vi "SVT Spurious Free Dynamic Range.vi"   [LabVIEW 2017, in "SoundVib_SingleTone.lvlib"]
doc: "Computes the spurious-free dynamic range (SFDR) of <B>scaled signal</B> and returns the detected fundamental frequency, detected fundamental amplitude, spurious free dynamic range, and all detected peaks. Wire data to the <B>scaled signal [EU]</B> input to determine the polymorphic instance to use or manually select the instance."
uses:
  <vilib>/addons/Sound and Vibration/svt_Single Tone Measurements/SoundVib_SingleTone.lvlib
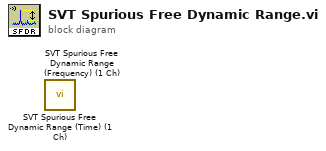
[diagram p0: block diagram]
diagram:
  n1 = call <vilib>:"SVT Spurious Free Dynamic Range (Time) (1 Ch).vi"() -> ()  [unwired: 12 in, 8 out]
  n2 = call <vilib>:"SVT Spurious Free Dynamic Range (Frequency) (1 Ch).vi"() -> ()  [unwired: 12 in, 8 out]
